vi "Legend.vi"(8 "error in (no error)":errorcluster, 10 "Plot labels":string[](array[string]), 11 "ITX Commands in":refnum<class "ITX Commands.lvclass">) -> (0 "error out":errorcluster, 3 "ITX Commands out":refnum<class "ITX Commands.lvclass">)   [LabVIEW 2019, in "ITX Commands.lvclass"]
uses:
  ITX Commands.lvclass
panel:
  out "resulting string":string
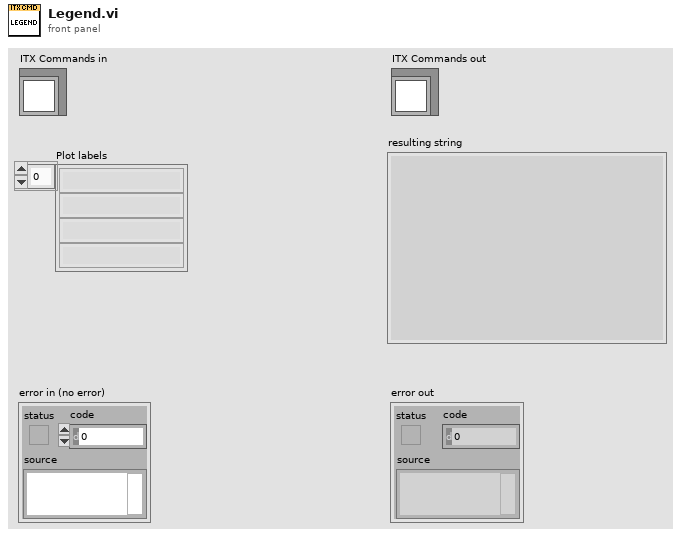
[diagram p1: front panel]
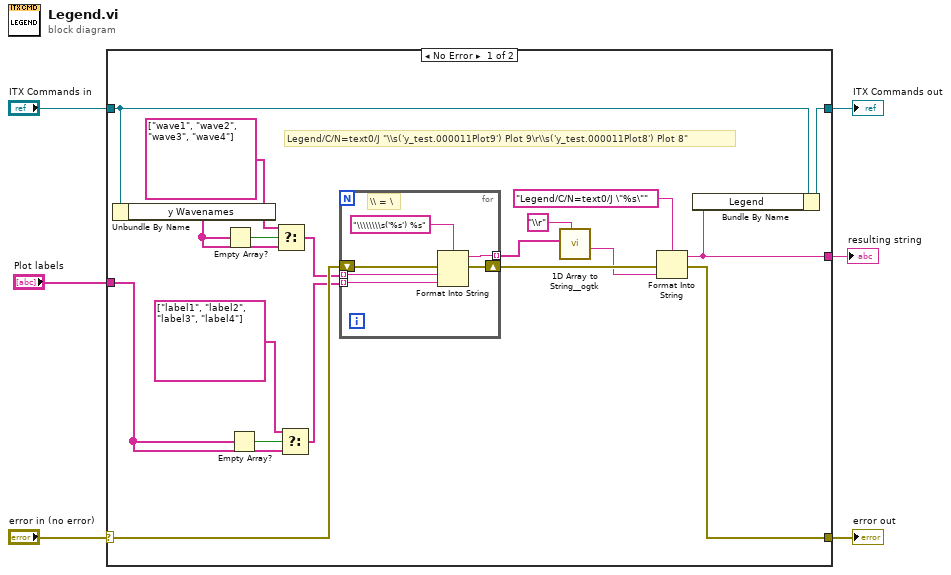
[diagram p0: block diagram]
diagram:
  n1 = case shown="No Error" "error in (no error)" {
    selector: "error in (no error)" -> [w17 w32]
    tunnel: [w11 w32] -> w5
    tunnel: [w24 w31] -> w3
    tunnel: "ITX Commands in" -> [w23 w31]
    tunnel: "Plot labels" -> [w8 _]
    tunnel: [w12 _] -> w1
    frame No Error {
      # "Legend/C/N=text0/J \"\\\\s('y_test.000011Plot9') Plot 9\\r\\\\s('y_test.000011Plot8') Plot 8\""
      n2 = Unbundle By Name(w23) -> ("y Wavenames"=w15:string[])
      n3 = Empty Array?(array=w15) -> (empty?=w16:bool)
      n4 = Empty Array?(array=w8) -> (empty?=w10:bool)
      n5 = Select(t=string[] ["wave1", "wave2", "wave3", "wave4"] ("y Wavenames"), s=w16, f=w15) -> (s? t:f=w14:string[])
      n6 = Select(t=string[] ["label1", "label2", "label3", "label4"] ("y Wavenames"), s=w10, f=w8) -> (s? t:f=w7:string[])
      n7 = for {
        tunnel: w14 -> [w27] mode=indexing
        shift-right: [w30] -> w21
        shift-left: w17 -> [w29]
        tunnel: w7 -> [w26] mode=indexing
        tunnel: [w25] -> w19 mode=indexing
        # "\\\\ = \\"
        n8 = Format Into String(format string="\\\\\\\\s('%s') %s", error in=w29, w27, w26) -> (resulting string=w25:string, error out=w30:errorcluster)  [unwired: 1 in]
      }
      n9 = call "1D Array to String__ogtk.vi"("delimiter (Tab)"="\\r", "Array of Strings"=w19) -> ("delimited string"=w18:string)  [unwired: 9 in]
      n10 = Format Into String(format string="Legend/C/N=text0/J \"%s\"", error in=w21, w18) -> (resulting string=w12:string, error out=w11:errorcluster)  [unwired: 1 in]
      n11 = Bundle By Name(cluster=w23, "Legend"=w12) -> (w24:refnum<class "ITX Commands.lvclass">)
    }
    frame Error {
    }
  }
  "error out" <- w5
  "ITX Commands out" <- w3
  "resulting string" <- w1
